vi "Digital Pattern Gen 1.0 Run.vi"(8 "error in (no error)":errorcluster, 11 "rt data in":T1 {"Compiled Data"."1.1 APUs"."shared settings"."cycle start" format="%#.15g"; "Compiled Data"."1.0 APUs"."shared settings"."cycle start" format="%#.15g"}) -> (0 "error out":errorcluster, 3 "rt data out":T1 {"Compiled Data"."1.1 APUs"."shared settings"."cycle start" format="%#.15g"; "Compiled Data"."1.0 APUs"."shared settings"."cycle start" format="%#.15g"})   [LabVIEW 2013, in "Engine Simulation Toolkit Engine.lvlib"]
uses:
  Engine Simulation Toolkit Engine.lvlib
  RT Data.ctl
  Shared/Compiled Data.ctl
  Shared/Engine Init Data.ctl
  Shared/1.0 APU Engine Data.ctl
  Shared/1.0 APU Engine FIFO Idxs.ctl
  Shared/Engine Status Data.ctl
  Shared/1.0 Analog Replay Engine Data.ctl
  Shared/1.0 Analog Replay FIFO Idxs.ctl
  Shared/1.0 Digital Pattern Gen Engine Data.ctl
  Shared/1.0 Digital Pattern Gen FIFO Idxs.ctl
  Shared/1.0 Event Timing Capture Engine Data.ctl
  Shared/1.0 Event Timing Capture FIFO Idxs.ctl
  Shared/1.0 Event Timing Measure Engine Data.ctl
  Shared/1.0 Event Timing Measure FIFO Idxs.ctl
  Shared/1.0 Knock Sensor Engine Data.ctl
  Shared/1.0 Knock Sensor FIFO Idxs.ctl
  Shared/1.0 Knock Cylinder Engine Data.ctl
  Shared/1.0 Knock Cylinder FIFO Idxs.ctl
  Shared/1.0 Directional Speed Engine Data.ctl
  Shared/1.0 Directional Speed FIFO Idxs.ctl
  Shared/1.1 APU Engine Data.ctl
  Shared/1.1 Event Timing Measure Engine Data.ctl
  Shared/1.3 Digital Pattern Gen Engine Data.ctl
  Shared/1.3 Digital Pattern Gen FIFO Idxs.ctl
  Shared/Bitfile EST Version.ctl
  Shared/1.3 APU Engine Data.ctl
  FPGA Refs.ctl
  APU 1.0 Run Refs.ctl
  APU 1.0 Output Ref.ctl
  APU 1.0 Input Ref.ctl
  Analog Replay 1.0 Input Ref.ctl
  Digital Pattern Gen 1.0 Input Ref.ctl
  Event Timing Capture 1.0 Output Ref.ctl
  Event Timing Measure 1.0 Output Ref.ctl
  Knock Cylinder 1.0 Input Ref.ctl
  Knock Sensor 1.0 Input Ref.ctl
  Directional Speed 1.0 Input Ref.ctl
  Digital Pattern Gen 1.3 Run Refs.ctl
  Digital Pattern Gen 1.3 Settings Ref.ctl
  Digital Pattern Gen 1.0 Write Inputs.vi
  Digital Pattern Gen 1.0 FPGA Inputs Write Node.vi
  Shared/Engine Simulation Toolkit Shared.lvlib
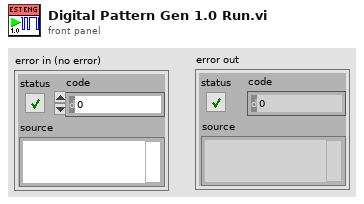
[diagram p1: front panel]
types:
  T1 = typedef "Engine Simulation Toolkit Engine.lvlib/RT Data.ctl" = cluster{"Compiled Data":T2, "FPGA Refs":T27}
  T2 = typedef "Engine Simulation Toolkit Shared.lvlib/Compiled Data.ctl" = cluster{"Init":T3, "1.0 APUs":T4[], "Status":T6, "DevOutFIFO":refnum<k33>, "DevInFIFO":refnum<k33>, "Device Inputs":dbl[], "Device Outputs":dbl[], "Last Device Inputs":dbl[], "1.0 Analog Replays":T7[], "Unused Analog Replays":string[], "1.0 Digital Pattern Gens":T9[], "Unused Digital Pattern Gens":string[], "1.0 Event Captures":T11[], "1.0 Event Measures":T13[], "1.0 Knock Sensors":T15[], "1.0 Knock Cylinders":T17[], "1.0 Directional Speed":T19[], "Unused Directional Sensors":string[], "1.1 APUs":T21[], "1.1 Event Measures":T22[], "1.3 Digital Pattern Gens":T23[], "Bitfile EST Version":T25, "1.3 APUs":T26[]}
  T3 = typedef "Engine Simulation Toolkit Shared.lvlib/Engine Init Data.ctl" = cluster{"CPU":i32, "RIO Address":string, "Decimation":i64, "Priority":i32, "Name":string, "Bitfile Path":path, "Input FIFO Size":i32, "Output FIFO Size":i32}
  T4 = typedef "Engine Simulation Toolkit Shared.lvlib/1.0 APU Engine Data.ctl" = cluster{"register names":cluster{"shared settings":string, "input":string, "settings":string, "output":string}, "shared settings":cluster{"cycle start":fxp<+,2,2>, "crank start":u16, "stuck limit":fxp<+,18,18>}, "settings":cluster{"acceleration":fxp<+,18,-20>, "max cycle":fxp<+,2,2>, "enable accel":bool}, "FIFO indexes":T5, "input":cluster{"desired speed":fxp<+/-,23,2>, "reset":bool}, "degrees of 1 cycle u16":dbl, "degrees of 1 crank u16":dbl}
  T5 = typedef "Engine Simulation Toolkit Shared.lvlib/1.0 APU Engine FIFO Idxs.ctl" = cluster{"inputs":cluster{"desired speed":i32, "reset":i32}, "outputs":cluster{"crank angle":i32, "cycle angle":i32, "actual speed":i32}}
  T6 = typedef "Engine Simulation Toolkit Shared.lvlib/Engine Status Data.ctl" = cluster{"FIFO indexes":cluster{"code":i32, "loop duration":i32, "late count":i32}}
  T7 = typedef "Engine Simulation Toolkit Shared.lvlib/1.0 Analog Replay Engine Data.ctl" = cluster{"register names":cluster{"load input":string, "settings":string, "input":string}, "settings":cluster{"ReverseNegate":bool, "CycleAngle":bool, "SpeedThreshold":fxp<+/-,23,2>, "AOBelowThreshold":i16}, "FIFO indexes":T8, "input":cluster{"Offset":i16, "VScaleSlope":fxp<+,18,6>, "VScaleIntercept":fxp<+/-,18,3>}, "offset convert":dbl, "DAC LUT":i16[], "SE_VScaleIntercept":fxp<+/-,18,3>, "SE_VScaleSlope":fxp<+,18,6>, "VOverride":bool, "ResetVolts":bool}
  T8 = typedef "Engine Simulation Toolkit Shared.lvlib/1.0 Analog Replay FIFO Idxs.ctl" = cluster{"enable voltage":i32, "volt slope":i32, "volt intercept":i32, "offset":i32}
  T9 = typedef "Engine Simulation Toolkit Shared.lvlib/1.0 Digital Pattern Gen Engine Data.ctl" = cluster{"register names":cluster{"load input":string, "settings":string, "input":string}, "settings":cluster{"edge 1":u16, "edge 2":u16, "cycle angle":bool, "enabled":bool, "first falling":bool}, "FIFO indexes":T10, "input":cluster{"Offset":i16}, "offset convert":dbl, "Position LUT":u16[]}
  T10 = typedef "Engine Simulation Toolkit Shared.lvlib/1.0 Digital Pattern Gen FIFO Idxs.ctl" = cluster{"offset":i32}
  T11 = typedef "Engine Simulation Toolkit Shared.lvlib/1.0 Event Timing Capture Engine Data.ctl" = cluster{"register names":cluster{"output":string}, "FIFO indexes":T12, "degrees of 1 u16":dbl, "wrap":bool, "window min":u16, "duration convert":dbl, "default start":dbl, "default end":dbl, "ref angle":dbl}
  T12 = typedef "Engine Simulation Toolkit Shared.lvlib/1.0 Event Timing Capture FIFO Idxs.ctl" = cluster{"start angle":i32, "end angle":i32, "duration":i32}
  T13 = typedef "Engine Simulation Toolkit Shared.lvlib/1.0 Event Timing Measure Engine Data.ctl" = cluster{"register names":cluster{"settings":string, "output":string}, "settings":cluster{"max":u16, "min":u16, "active high":bool, "wrap":bool, "full window":bool}, "FIFO indexes":T14}
  T14 = typedef "Engine Simulation Toolkit Shared.lvlib/1.0 Event Timing Measure FIFO Idxs.ctl" = cluster{"stuck active":i32, "win all active":i32, "win orph start":i32, "win orph end":i32}
  T15 = typedef "Engine Simulation Toolkit Shared.lvlib/1.0 Knock Sensor Engine Data.ctl" = cluster{"register names":cluster{"settings":string, "input":string}, "settings":cluster{"low freq (periods/tick)":fxp<+,32,0>, "high freq (periods/tick)":fxp<+,32,0>, "duration (1.25MHz tics)":fxp<+,18,18>, "low freq speed slope":fxp<+,16,-3>, "low freq speed intercept":fxp<+,10,-10>, "low freq by speed":bool}, "DAC multiplier":dbl, "FIFO indexes":T16, "input":cluster{"low freq scaler":fxp<+,10,0>}}
  T16 = typedef "Engine Simulation Toolkit Shared.lvlib/1.0 Knock Sensor FIFO Idxs.ctl" = cluster{"amp":i32}
  T17 = typedef "Engine Simulation Toolkit Shared.lvlib/1.0 Knock Cylinder Engine Data.ctl" = cluster{"register names":cluster{"settings":string, "input":string}, "settings":cluster{"seed":u16, "reset":bool}, "input":cluster{"probability compare":u16, "high freq scaler":fxp<+,10,0>, "trigger position":u16}, "DAC multiplier":dbl, "FIFO indexes":T18, "Angle multiplier":dbl}
  T18 = typedef "Engine Simulation Toolkit Shared.lvlib/1.0 Knock Cylinder FIFO Idxs.ctl" = cluster{"prob":i32, "amp":i32, "pos":i32}
  T19 = typedef "Engine Simulation Toolkit Shared.lvlib/1.0 Directional Speed Engine Data.ctl" = cluster{"register names":cluster{"settings":string, "input":string, "load input":string}, "settings":cluster{"Upper Value":u16, "Lower Value":u16, "Upper Index":fxp<+,10,10>, "Lower Index":fxp<+,10,10>, "Enabled":bool}, "input":cluster{"td (tics)":u16, "tf (tics)":u16, "tr (tics)":u16}, "FIFO indexes":T20, "Tooth Centers LUT":u16[]}
  T20 = typedef "Engine Simulation Toolkit Shared.lvlib/1.0 Directional Speed FIFO Idxs.ctl" = cluster{"td":i32, "tf":i32, "tr":i32}
  T21 = typedef "Engine Simulation Toolkit Shared.lvlib/1.1 APU Engine Data.ctl" = cluster{"register names":cluster{"shared settings":string, "input":string, "settings":string, "output":string, "go":string}, "shared settings":cluster{"cycle start":fxp<+,2,2>, "crank start":u16, "stuck limit":fxp<+,18,18>}, "settings":cluster{"acceleration":fxp<+,18,-20>, "max cycle":fxp<+,2,2>, "enable accel":bool}, "FIFO indexes":T5, "input":cluster{"desired speed":fxp<+/-,23,2>, "reset":bool}, "degrees of 1 cycle u16":dbl, "degrees of 1 crank u16":dbl}
  T22 = typedef "Engine Simulation Toolkit Shared.lvlib/1.1 Event Timing Measure Engine Data.ctl" = cluster{"register names":cluster{"settings":string, "output":string}, "settings":cluster{"max":u16, "min":u16, "active high":bool, "wrap":bool}, "FIFO indexes":T14}
  T23 = typedef "Engine Simulation Toolkit Shared.lvlib/1.3 Digital Pattern Gen Engine Data.ctl" = cluster{"register names":cluster{"load input":string, "settings":string, "input":string}, "settings":cluster{"edge 1":u16, "edge 2":u16, "cycle angle":bool, "enabled":bool, "first falling":bool, "fault":bool, "fault wrap":bool, "fault value":bool, "fault count":fxp<+,4,4>, "use fault count":bool}, "FIFO indexes":T24, "input":cluster{"Offset":i16}, "deg to u16 scale":dbl, "Position LUT":u16[], "# of teeth":i16, "max angle":dbl}
  T24 = typedef "Engine Simulation Toolkit Shared.lvlib/1.3 Digital Pattern Gen FIFO Idxs.ctl" = cluster{"offset":i32, "command":i32, "rotations":i32, "start angle":i32, "stop angle":i32, "tooth to rem":i32, "trigger":i32, "valid":i32}
  T25 = typedef "Engine Simulation Toolkit Shared.lvlib/Bitfile EST Version.ctl" = enum16{"1.0", "1.1", "1.2", "1.3"}
  T26 = typedef "Engine Simulation Toolkit Shared.lvlib/1.3 APU Engine Data.ctl" = cluster{"register names":cluster{"shared settings":string, "input":string, "settings":string, "output":string, "go":string}, "shared settings":cluster{"start":fxp<+,17,17>, "stuck limit":fxp<+,18,18>}, "settings":cluster{"acceleration":fxp<+,18,-20>, "enable accel":bool}, "FIFO indexes":T5, "input":cluster{"desired speed":fxp<+/-,23,2>, "reset":bool}, "degrees of 1 cycle u16":dbl, "degrees of 1 crank u16":dbl}
  T27 = typedef "Engine Simulation Toolkit Engine.lvlib/FPGA Refs.ctl" = cluster{"1.0 APUs":T28[], "FPGA ref":refnum<k20>, "1.0 Analog Replays":T31[], "1.0 Dig Pat Gens":T32[], "1.0 Event Captures":T33[], "1.0 Event Measures":T34[], "1.0 Knock Cylinders":T35[], "1.0 Knock Sensors":T36[], "1.0 Directional Speed Sensors":T37[], "1.3 Dig Pat Gens":T38[]}
  T28 = typedef "Engine Simulation Toolkit Engine.lvlib/APU 1.0 Run Refs.ctl" = cluster{"output reference":T29, "input reference":T30}
  T29 = typedef "Engine Simulation Toolkit Engine.lvlib/APU 1.0 Output Ref.ctl" = refnum<k20>
  T30 = typedef "Engine Simulation Toolkit Engine.lvlib/APU 1.0 Input Ref.ctl" = refnum<k20>
  T31 = typedef "Engine Simulation Toolkit Engine.lvlib/Analog Replay 1.0 Input Ref.ctl" = refnum<k20>
  T32 = typedef "Engine Simulation Toolkit Engine.lvlib/Digital Pattern Gen 1.0 Input Ref.ctl" = refnum<k20>
  T33 = typedef "Engine Simulation Toolkit Engine.lvlib/Event Timing Capture 1.0 Output Ref.ctl" = refnum<k20>
  T34 = typedef "Engine Simulation Toolkit Engine.lvlib/Event Timing Measure 1.0 Output Ref.ctl" = refnum<k20>
  T35 = typedef "Engine Simulation Toolkit Engine.lvlib/Knock Cylinder 1.0 Input Ref.ctl" = refnum<k20>
  T36 = typedef "Engine Simulation Toolkit Engine.lvlib/Knock Sensor 1.0 Input Ref.ctl" = refnum<k20>
  T37 = typedef "Engine Simulation Toolkit Engine.lvlib/Directional Speed 1.0 Input Ref.ctl" = refnum<k20>
  T38 = typedef "Engine Simulation Toolkit Engine.lvlib/Digital Pattern Gen 1.3 Run Refs.ctl" = cluster{"input":T32, "settings":T39}
  T39 = typedef "Engine Simulation Toolkit Engine.lvlib/Digital Pattern Gen 1.3 Settings Ref.ctl" = refnum<k20>
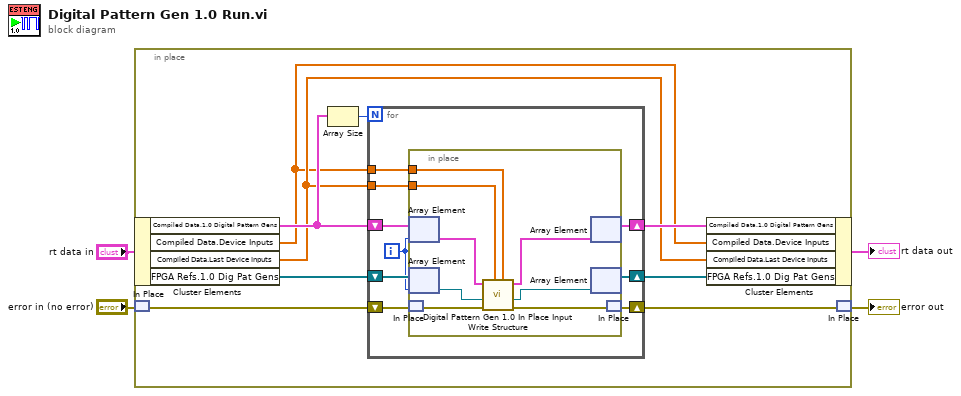
[diagram p0: block diagram]
diagram:
  n1 = in-place {
    n2 = in-place-cluster #1("rt data in") -> ("Compiled Data.1.0 Digital Pattern Gens"=w11:T9[], "Compiled Data.Device Inputs"=w7:dbl[], "Compiled Data.Last Device Inputs"=w8:dbl[], "FPGA Refs.1.0 Dig Pat Gens"=w6:T32[])
    n3 = in-place-match #2("error in (no error)") -> (w13:errorcluster)
    n4 = Array Size(array=w11) -> (size(s)=w12:i32)
    n5 = for {
      N: w12 -> [_]
      shift-right: [w19] -> w9
      shift-left: w11 -> [w20]
      shift-right: [w21] -> w10
      shift-left: w13 -> [w22]
      tunnel: w8 -> [w18]
      tunnel: w7 -> [w17]
      shift-right: [w15] -> w5
      shift-left: w6 -> [w16]
      i -> [w14]
      n6 = in-place {
        in-place-border: w18 -> [w27]
        in-place-border: w17 -> [w26]
        n7 = in-place-array #3(w20, w14) -> (w23:T9)
        n8 = in-place-array #4(w16, w14) -> (w25:T32)
        n9 = in-place-match #5(w22) -> (w30:errorcluster)
        n10 = call "Digital Pattern Gen 1.0 In Place Input Write Structure.vi"("Device Inputs"=w26, "Last Device Inputs"=w27, "error in (no error)"=w30, "FPGA ref in"=w25, "1.0 Digital Pattern Gen in"=w23) -> ("error out"=w29:errorcluster, "FPGA ref out"=w24:T32, "1.0 Digital Pattern Gen out"=w28:T9)  [unwired: 4 in]
        n11 = in-place-array #3(w28) -> (w19:T9[])  [unwired: 1 out]
        n12 = in-place-array #4(w24) -> (w15:T32[])  [unwired: 1 out]
        n13 = in-place-match #5(w29) -> (w21:errorcluster)
      }
    }
    n14 = in-place-cluster #1("Compiled Data.1.0 Digital Pattern Gens"=w9, "Compiled Data.Device Inputs"=w7, "Compiled Data.Last Device Inputs"=w8, "FPGA Refs.1.0 Dig Pat Gens"=w5) -> (→"rt data out":T1)
    n15 = in-place-match #2(w10) -> (→"error out":errorcluster)
  }
